vi "Set Laser PWM.vi"(8 "error in (no error)":errorcluster, 10 "PWM Duty cycle":u8, 11 "VISA Refnum in":refnum<visa-resource-name>) -> (0 "error out":errorcluster, 3 "VISA Refnum out":refnum<visa-resource-name>)   [LabVIEW 2020, in "Control de MaP.lvlib"]
uses:
  Write--command.vi
  Control de MaP.lvlib
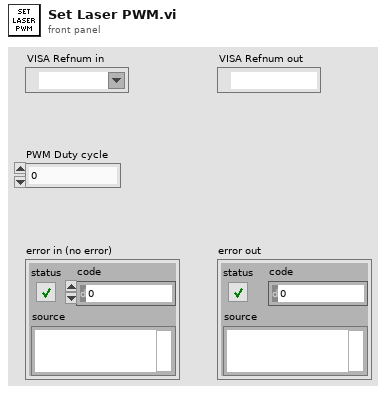
[diagram p1: front panel]
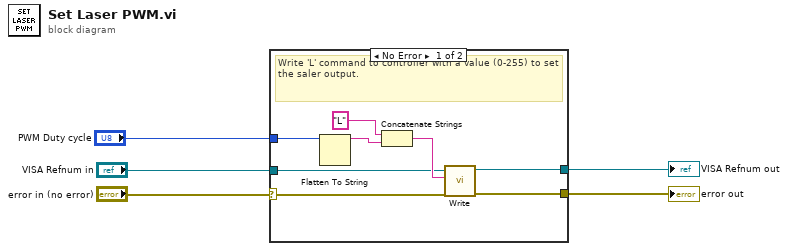
[diagram p0: block diagram]
diagram:
  n1 = case shown="No Error" "error in (no error)" {
    selector: "error in (no error)" -> [w6 w14]
    tunnel: "PWM Duty cycle" -> [w10 _]
    tunnel: [w9 w15] -> w4
    tunnel: "VISA Refnum in" -> [w8 w15]
    tunnel: [w7 w14] -> w2
    frame No Error {
      # "Write 'L' command to controller with a value (0-255) to set the saler output."
      n2 = Flatten To String(anything=w10) -> (data string=w12:string)  [unwired: 3 in, 2 out]
      n3 = Concatenate Strings("L" ("Command"), w12) -> (w13:string)
      n4 = call-poly "Write.vi"("error in (no error)"=w6, "Command"=w13, "VISA resource name"=w8) -> ("error out"=w7:errorcluster, "VISA resource name out"=w9:refnum<visa-resource-name>)  [unwired: 6 in, 1 out]
    }
    frame Error {
    }
  }
  "VISA Refnum out" <- w4
  "error out" <- w2
